vi "Reference_Data_Read.vi"(6 "Active Sensors":bool[](array[boolean]), 7 "chkeach_ch":bool, 8 "error in":errorcluster caption="错误输入", 9 "PDLSTS":refnum<k24>, 10 "Data_struct":refnum<k24>[](array[refnum]), 11 "TSL":refnum<k24>) -> (0 "error IO":errorcluster)   [LabVIEW 2017]
doc: "// Reference Data Read\n// This function must use after \"SET\""
uses:
  D:/test/PDLSTS/LV_PDL_Sample/DLL/STSProcess.dll
  DLL/STSProcess.dll
  D:/test/PDLSTS/LV_PDL_Sample/DLL/InstrumentDLL.dll
  DLL/InstrumentDLL.dll
  <vilib>/Utility/file.llb/Read Delimited Spreadsheet (string).vi
panel:
  in  "txtstepwave":dbl caption="WavelengthStep(nm)"
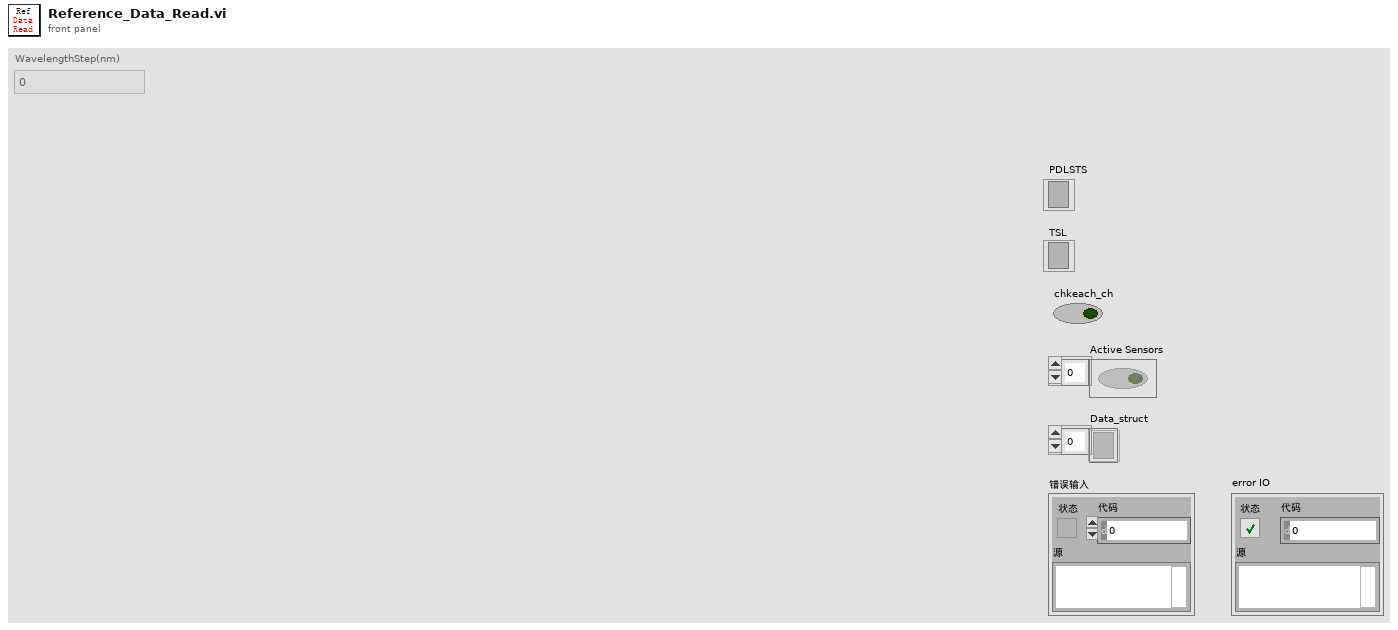
[diagram p1: front panel]
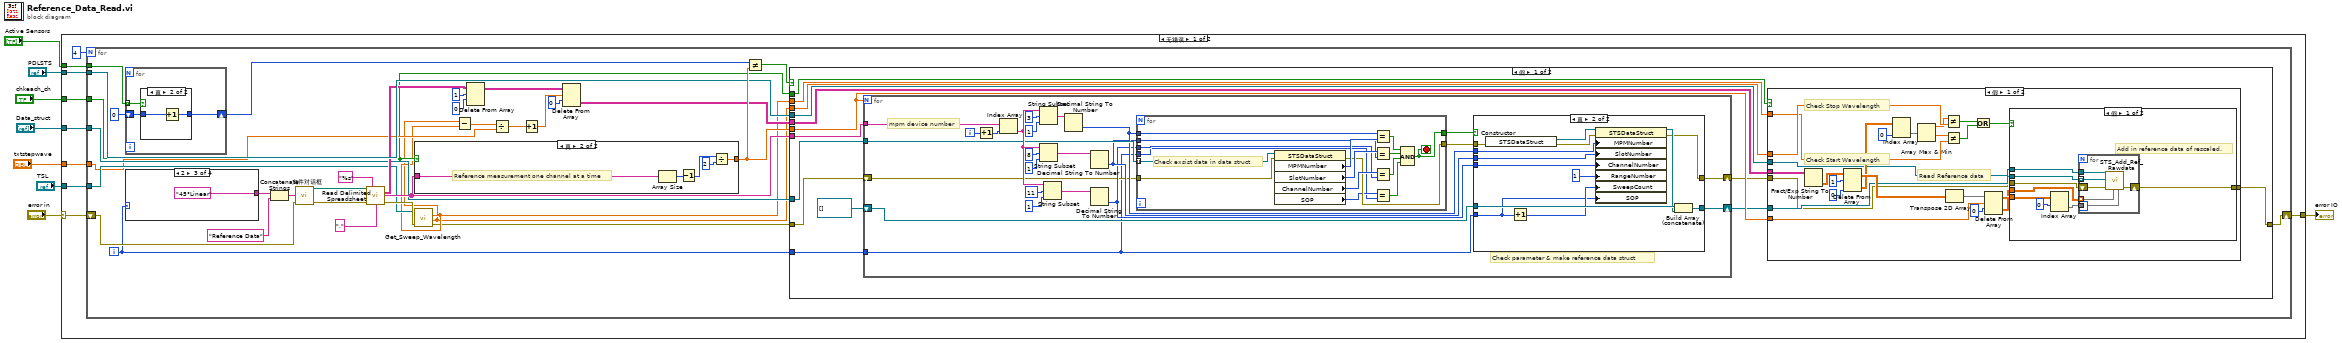
[diagram p0: block diagram]
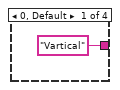
[diagram p2: hidden frame]
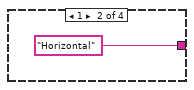
[diagram p3: hidden frame]
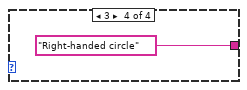
[diagram p4: hidden frame]
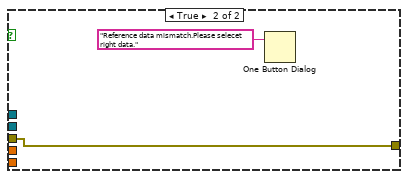
[diagram p5: hidden frame]
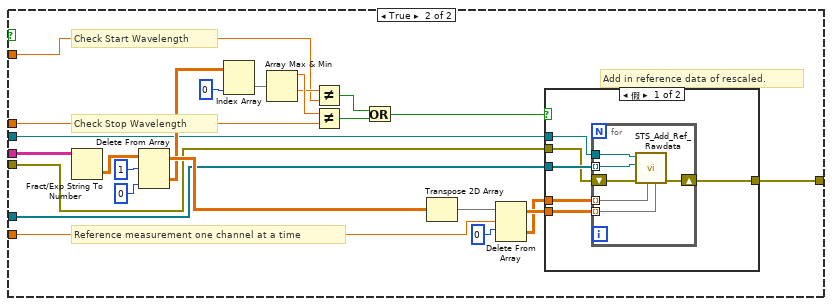
[diagram p6: hidden frame]
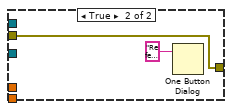
[diagram p7: hidden frame]
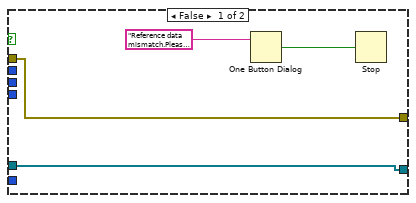
[diagram p8: hidden frame]
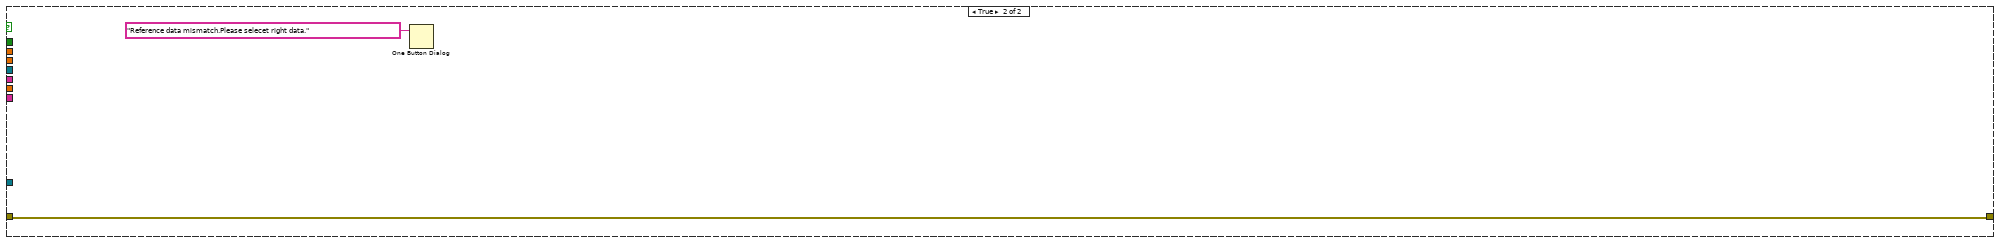
[diagram p9: hidden frame]
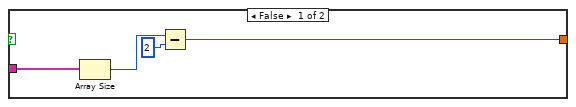
[diagram p11: hidden frame]
diagram:
  n1 = case shown="无错误" "error in" {
    selector: "error in" -> [w16 w222]
    tunnel: "PDLSTS" -> [w17 _]
    tunnel: [w15 w222] -> w6
    tunnel: "Data_struct" -> [w14 _]
    tunnel: "TSL" -> [w13 _]
    tunnel: "Active Sensors" -> [w12 _]
    tunnel: "txtstepwave" -> [w11 _]
    tunnel: "chkeach_ch" -> [w10 _]
    frame No Error {
      n2 = for {
        N: 4 -> [_]
        tunnel: w17 -> [w45]
        tunnel: w14 -> [w35]
        tunnel: w13 -> [w34]
        tunnel: w12 -> [w33]
        tunnel: w11 -> [w32]
        tunnel: w10 -> [w31]
        shift-right: [w37] -> w15
        shift-left: w16 -> [w38]
        i -> [w18]
        n3 = for {
          shift-right: [w208] -> w48
          shift-left: 0 -> [w209]
          tunnel: w33 -> [w207] mode=indexing
          n4 = case shown="真" w207 {
            tunnel: w209 -> [w210 w212]
            tunnel: [w210 w211] -> w208
            frame False {
            }
            frame True {
              n5 = Increment(x=w212) -> (x+1=w211:i32)
            }
          }
        }
        n6 = case shown="2" w18 {
          tunnel: ["Vartical" "Horizontal" "45°Linear" "Right-handed circle"] -> w21
          frame 0, Default {
          }
          frame 1 {
          }
          frame 2 {
          }
          frame 3 {
          }
        }
        n7 = Concatenate Strings(w21, "Reference Data" ("default name")) -> (w19:string)
        n8 = call "文件对话框"("default name"=w19, "error in"=w38) -> ("selected path"=w49:path, "error out"=w50:errorcluster)  [unwired: 10 in, 2 out]
        n9 = call-poly <vilib>:"Read Delimited Spreadsheet.vi"("file path (dialog if empty)"=w49, "format (%s)"="%s", "error in (no error)"=w50, "delimiter (\\t)"="," ("delimiter (\\t)")) -> ("all rows"=w40:string[][], "first row"=w51:string[], "error out"=w36:errorcluster)  [unwired: 6 in, 3 out]
        n10 = case shown="真" w31 {
          tunnel: w51 -> [w216 w221]
          tunnel: [w214 w218] -> w46
          frame False {
            n11 = Array Size(array=w216) -> (size(s)=w213:i32)
            n12 = Subtract(x=w213, y=2) -> (x-y=w214:i32)
          }
          frame True {
            # "Reference measurement one channel at a time"
            n13 = Array Size(array=w221) -> (size(s)=w217:i32)
            n14 = Decrement(x=w217) -> (x-1=w220:i32)
            n15 = Divide(x=w220, y=2) -> (x/y=w218:dbl)
          }
        }
        n16 = call "Get_Sweep_Wavelength.vi"("error in (no error)"=w36, ".NET Reference in"=w34) -> ("error out"=w22:errorcluster, "endwave out"=w23:dbl, "startwave out"=w24:dbl)  [unwired: 6 in, 1 out]
        n17 = Subtract(x=w23, y=w24) -> (x-y=w29:dbl)
        n18 = Delete From Array(array=w40, length=1 ("长度"), index (row)=0 ("索引 (行)")) -> (array with subset deleted=w39:string[][])  [unwired: 1 in, 1 out]
        n19 = Divide(x=w29, y=w32) -> (x/y=w28:dbl)
        n20 = Increment(x=w28) -> (x+1=w27:dbl)
        n21 = Delete From Array(array=w39, length=w27, index (row)=0 ("索引 (行)")) -> (deleted portion=w25:string[][])  [unwired: 1 in, 1 out]
        n22 = Not Equal?(x=w48, y=w46) -> (x != y?=w30:bool)
        n23 = case shown="假" w30 {
          tunnel: w46 -> [w69 _]
          tunnel: w51 -> [w68 _]
          tunnel: w35 -> [w67 _]
          tunnel: w31 -> [w66 _]
          tunnel: w25 -> [w65 _]
          tunnel: w23 -> [w64 _]
          tunnel: w45 -> [w61 _]
          tunnel: w24 -> [w63 _]
          tunnel: [w59 w205] -> w37
          tunnel: w22 -> [w58 w205]
          tunnel: w18 -> [w56 _]
          frame False {
            n24 = for {
              N: w69 -> [_]
              tunnel: w68 -> [w171]
              tunnel: w67 -> [w161]
              shift-right: [w153] -> w60
              shift-left: refnum<k24>[] [] ("Data_struct") -> [w152]
              shift-right: [w149] -> w57
              shift-left: w58 -> [w151]
              tunnel: w56 -> [w148]
              i -> [w166]
              # "Check parameter & make reference data struct"
              # "mpm device number"
              n25 = Increment(x=w166) -> (x+1=w165:i32)
              n26 = Index Array(array=w171, index=w165) -> (element=w162:string)
              n27 = String Subset(string=w162, offset (0)=3 ("偏移量(0)"), length (rest)=1 ("长度（剩余）")) -> (substring=w158:string)
              n28 = String Subset(string=w162, offset (0)=8 ("偏移量(0)"), length (rest)=1 ("长度（剩余）")) -> (substring=w157:string)
              n29 = String Subset(string=w162, offset (0)=11 ("偏移量(0)"), length (rest)=1 ("长度（剩余）")) -> (substring=w159:string)
              n30 = Decimal String To Number(string=w158) -> (number=w156:i32)  [unwired: 2 in, 1 out]
              n31 = Decimal String To Number(string=w157) -> (number=w155:i32)  [unwired: 2 in, 1 out]
              n32 = Decimal String To Number(string=w159) -> (number=w154:i32)  [unwired: 2 in, 1 out]
              n33 = for {
                tunnel: w161 -> [w187] mode=indexing
                tunnel: [w172] -> w160
                tunnel: w154 -> [w180]
                tunnel: w156 -> [w179]
                tunnel: w155 -> [w178]
                tunnel: w151 -> [w177]
                tunnel: [w176] -> w150
                tunnel: w148 -> [w174]
                stop <- w172 stop-if-true
                # "Check exsist data in data struct"
                n34 = property on="属性节点" class="STSDataStruct"(reference=w187, error in=w177) -> (error out=w176:errorcluster, "MPMNumber"=w186:i32, "SlotNumber"=w185:i32, "ChannelNumber"=w184:i32, "SOP"=w175:i32)  [unwired: 1 out]
                n35 = Equal?(x=w179, y=w186) -> (x = y?=w183:bool)
                n36 = Equal?(x=w185, y=w178) -> (x = y?=w182:bool)
                n37 = Equal?(x=w184, y=w180) -> (x = y?=w181:bool)
                n38 = Equal?(x=w175, y=w174) -> (x = y?=w173:bool)
                n39 = Compound Arithmetic op=AND ("复合运算")(w183, w182, w181, w173) -> (w172:bool)
              }
              n40 = case shown="真" w160 {
                tunnel: w156 -> [_ w204]
                tunnel: w155 -> [_ w203]
                tunnel: w154 -> [_ w202]
                tunnel: w152 -> [w190 w201]
                tunnel: [w190 w199] -> w153
                tunnel: w150 -> [w188 w196]
                tunnel: [w188 w195] -> w149
                tunnel: w148 -> [_ w192]
                frame False {
                  n41 = One Button Dialog(message="Reference data mismatch.Please selecet right data." ("消息")) -> (true=w189:bool)  [unwired: 1 in]
                  n42 = Stop(stop? (T)=w189) -> ()
                }
                frame True {
                  n43 = constructor class="STSDataStruct"(error in=w196) -> (reference out=w198:refnum<k24>, error out=w197:errorcluster)  [unwired: 2 in, 1 out]
                  n44 = Increment(x=w192) -> (x+1=w194:i32)
                  n45 = property on="属性节点" class="STSDataStruct"(reference=w198, error in=w197, "MPMNumber"=w204, "SlotNumber"=w203, "ChannelNumber"=w202, "RangeNumber"=1, "SweepCount"=w194, "SOP"=w192) -> (reference out=w200:refnum<k24>, error out=w195:errorcluster)
                  n46 = Build Array (concatenate)(w201, w200) -> (w199:refnum<k24>[])
                }
              }
            }
            n47 = case shown="假" w66 {
              tunnel: w65 -> [w79 w119]
              tunnel: w69 -> [w82 w122]
              tunnel: w64 -> [w93 w133]
              tunnel: w63 -> [w80 w120]
              tunnel: w60 -> [w75 w112]
              tunnel: w61 -> [w72 w115]
              tunnel: [w71 w110] -> w59
              tunnel: w57 -> [w70 w111]
              frame False {
                # "Check Stop Wavelength"
                # "Check Start Wavelength"
                # "Read Reference data"
                n48 = Fract/Exp String To Number(string=w79) -> (number=w92:dbl[][])  [unwired: 3 in, 1 out]
                n49 = Delete From Array(array=w92, length=1 ("长度"), index (col)=0 ("禁用的索引 (列)")) -> (deleted portion=w88:dbl[][], array with subset deleted=w89:dbl[][])  [unwired: 1 in]
                n50 = Index Array(array=w88, index (col)=0 ("禁用的索引 (列)")) -> (element=w86:dbl[])  [unwired: 1 in]
                n51 = Array Max & Min(array=w86) -> (max value=w85:dbl, min value=w84:dbl)  [unwired: 2 out]
                n52 = Not Equal?(x=w85, y=w93) -> (x != y?=w78:bool)
                n53 = Not Equal?(x=w84, y=w80) -> (x != y?=w77:bool)
                n54 = Transpose 2D Array(2D array=w89) -> (transposed array=w83:dbl[][])
                n55 = Or(x=w78, y=w77) -> (x .or. y?=w76:bool)
                n56 = Delete From Array(array=w83, length=w82, index (row)=0 ("索引 (行)")) -> (deleted portion=w73:dbl[][], array with subset deleted=w74:dbl[][])  [unwired: 1 in]
                n57 = case shown="假" w76 {
                  tunnel: w72 -> [w101 _]
                  tunnel: w75 -> [w100 _]
                  tunnel: w74 -> [w98 _]
                  tunnel: w73 -> [w99 _]
                  tunnel: [w95 w108] -> w71
                  tunnel: w70 -> [w94 w108]
                  frame False {
                    # "Add in reference data of rescaled."
                    n58 = Index Array(array=w98, index (row)=0 ("索引 (行)")) -> (element=w96:dbl[])  [unwired: 1 in]
                    n59 = for {
                      tunnel: w101 -> [w107]
                      tunnel: w100 -> [w106] mode=indexing
                      tunnel: w99 -> [w105] mode=indexing
                      tunnel: w96 -> [w104]
                      shift-right: [w103] -> w95
                      shift-left: w94 -> [w102]
                      n60 = call "STS_Add_Ref_Rawdata.vi"("monitorData"=w104, "MPMData"=w105, "错误输入（无错误）"=w102, "Setting"=w106, "STSProcess.PDLSTS"=w107) -> ("错误输出"=w103:errorcluster)  [unwired: 5 in, 1 out]
                    }
                  }
                  frame True {
                    n61 = One Button Dialog(message="Reference data mismatch.Please selecet right data." ("消息")) -> ()  [unwired: 1 in, 1 out]
                  }
                }
              }
              frame True {
                # "Add in reference data of rescaled."
                # "Check Stop Wavelength"
                # "Check Start Wavelength"
                # "Reference measurement one channel at a time"
                n62 = Fract/Exp String To Number(string=w119) -> (number=w132:dbl[][])  [unwired: 3 in, 1 out]
                n63 = Delete From Array(array=w132, length=1 ("长度"), index (col)=0 ("禁用的索引 (列)")) -> (deleted portion=w128:dbl[][], array with subset deleted=w129:dbl[][])  [unwired: 1 in]
                n64 = Index Array(array=w128, index (col)=0 ("禁用的索引 (列)")) -> (element=w126:dbl[])  [unwired: 1 in]
                n65 = Array Max & Min(array=w126) -> (max value=w125:dbl, min value=w124:dbl)  [unwired: 2 out]
                n66 = Not Equal?(x=w124, y=w120) -> (x != y?=w117:bool)
                n67 = Not Equal?(x=w125, y=w133) -> (x != y?=w118:bool)
                n68 = Or(x=w117, y=w118) -> (x .or. y?=w116:bool)
                n69 = Transpose 2D Array(2D array=w129) -> (transposed array=w123:dbl[][])
                n70 = Delete From Array(array=w123, length=w122, index (row)=0 ("索引 (行)")) -> (deleted portion=w113:dbl[][], array with subset deleted=w114:dbl[][])  [unwired: 1 in]
                n71 = case shown="假" w116 {
                  tunnel: w115 -> [w139 _]
                  tunnel: w112 -> [w138 _]
                  tunnel: w114 -> [w137 _]
                  tunnel: w113 -> [w136 _]
                  tunnel: w111 -> [w135 w146]
                  tunnel: [w134 w146] -> w110
                  frame False {
                    n72 = for {
                      tunnel: w139 -> [w145]
                      tunnel: w138 -> [w144] mode=indexing
                      tunnel: w137 -> [w143] mode=indexing
                      tunnel: w136 -> [w142] mode=indexing
                      shift-right: [w140] -> w134
                      shift-left: w135 -> [w141]
                      n73 = call "STS_Add_Ref_Rawdata.vi"("monitorData"=w143, "MPMData"=w142, "错误输入（无错误）"=w141, "Setting"=w144, "STSProcess.PDLSTS"=w145) -> ("错误输出"=w140:errorcluster)  [unwired: 5 in, 1 out]
                    }
                  }
                  frame True {
                    n74 = One Button Dialog(message="Reference data mismatch.Please selecet right data." ("消息")) -> ()  [unwired: 1 in, 1 out]
                  }
                }
              }
            }
          }
          frame True {
            n75 = One Button Dialog(message="Reference data mismatch.Please selecet right data." ("消息")) -> ()  [unwired: 1 in, 1 out]
          }
        }
      }
    }
    frame Error {
    }
  }
  "error IO" <- w6
